vi "Autonomous Independent.vi"   [LabVIEW 2013]
doc: "This VI is called when autonomous begins, and will automatically be terminated when autonomous ends. You can carry out timed or sensor driven robot movement independently without needing to return to the caller."
uses:
  Robot Global Data.vi
  <vilib>/Rock Robotics/WPI/Joystick/WPI_JoystickGetSetRefNum.vi
types:
  T1 = typedef "WPI_DigitalInputDevRef.ctl" = cluster{"DevStatus":errorcluster, "DIO Channel":T2, "Digital Module":T3}
  T2 = typedef "FPGA_DIOChannel.ctl" = enum8{"DIO 1", "DIO 2", "DIO 3", "DIO 4", "DIO 5", "DIO 6", "DIO 7", "DIO 8", "DIO 9", "DIO 10", "DIO 11", "DIO 12", "DIO 13", "DIO 14", "Invalid"}
  T3 = typedef "FPGA_TypedefDigitalModule.ctl" = enum16{"Digital Module 1", "Digital Module 2"}
  T4 = typedef "WPI_MotorControlDeviceRef.ctl" = cluster{"DeviceStatus":errorcluster, "Type":enum16{"PWM", "CAN"}, "PWM":cluster{"Digital Module":T3, "PWM Channel":T5, "DeadBand":T6}, "CAN":cluster{"Device Number":u8, "Control Mode":T7, "Semaphore":T8, "Max Vout":dbl}, "Invert":bool, "TransformRef":T9, "InvTransformRef":T9}
  T5 = typedef "FPGA_DIOPWMChannel.ctl" = enum8{"PWM 1", "PWM 2", "PWM 3", "PWM 4", "PWM 5", "PWM 6", "PWM 7", "PWM 8", "PWM 9", "PWM 10", "Invalid"}
  T6 = typedef "WPI_PWMDeadband.ctl" = cluster{"Name":string, "maxPositivePwm":i32, "minPositivePwm":i32, "centerPwm":i32, "maxNegativePwm":i32, "minNegativePwm":i32, "angularRange":u16}
  T7 = typedef "WPI_CANJaguar_ControlMode.ctl" = enum8{"Percent VBus", "Current", "Speed", "Position", "Voltage"}
  T8 = typedef "Semaphore RefNum" = refnum<k1>
  T9 = typedef "WPI_PWMTransform_ConPane.ctl" = refnum<vi>
  T10 = typedef "WPI_JoystickDevRef.ctl" = cluster{"Device":T11}
  T11 = typedef "WPI_JoystickDeviceEnum.ctl" = enum16{"USB 1", "USB 2", "USB 3", "USB 4", "Kinect 1", "Kinect 2"}
  T12 = cluster{"axis 1 (x)":dbl, "axis 2 (y)":dbl, "axis 3 (throttle)":dbl, "axis 4":dbl, "axis 5":dbl, "axis 6":dbl}
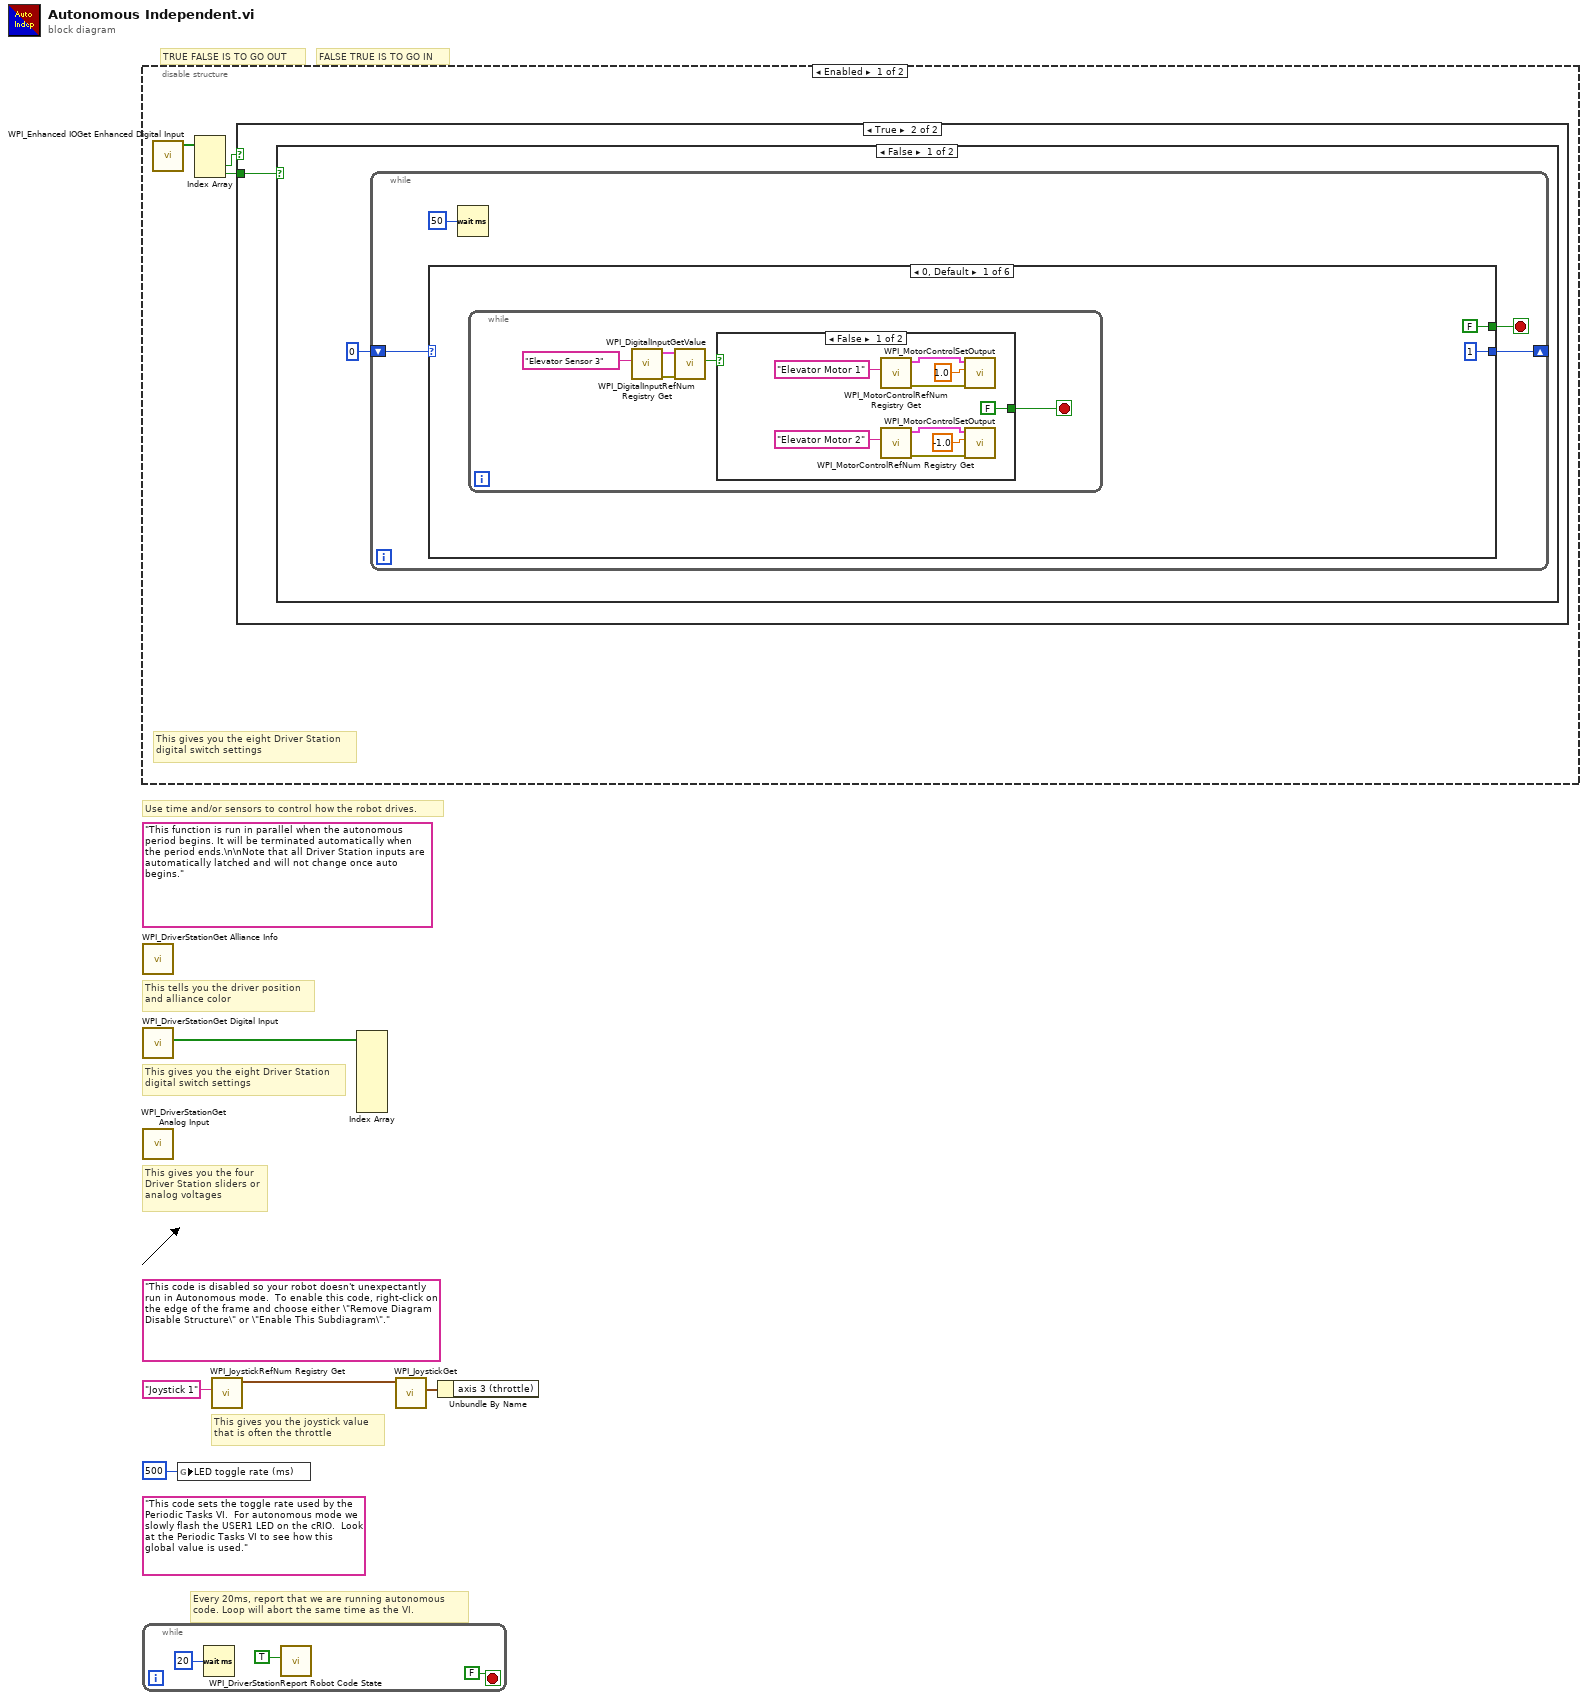
[diagram p0: block diagram]
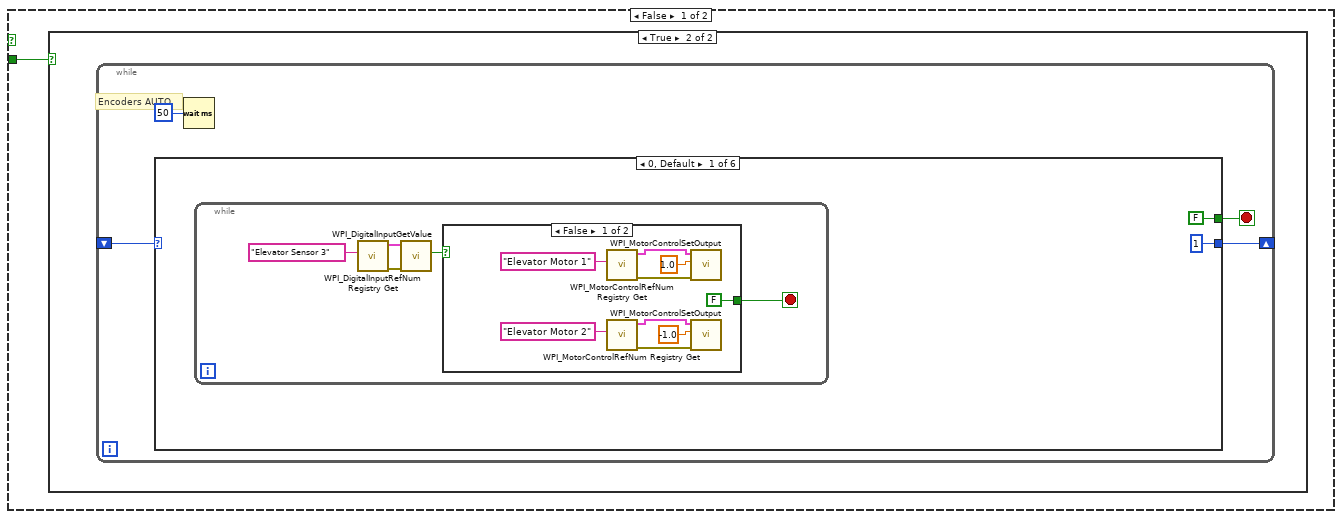
[diagram p2: hidden frame]
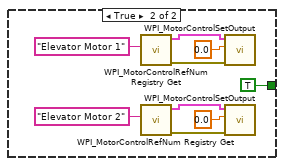
[diagram p4: hidden frame]
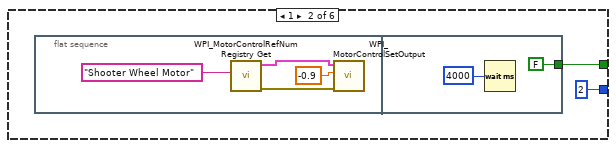
[diagram p5: hidden frame]
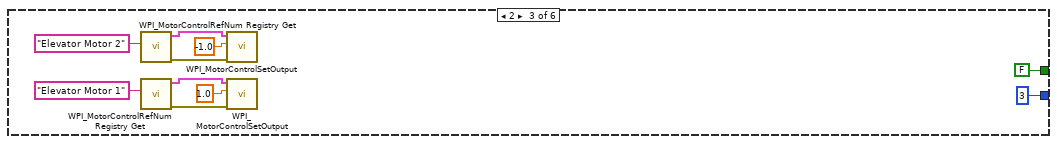
[diagram p6: hidden frame]
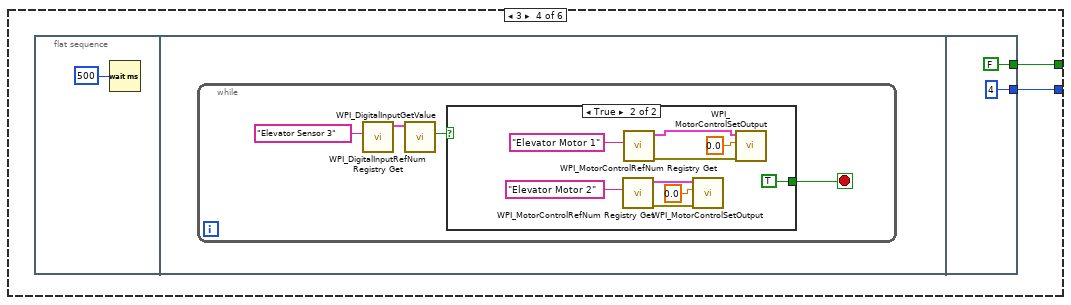
[diagram p7: hidden frame]
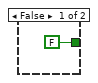
[diagram p8: hidden frame]
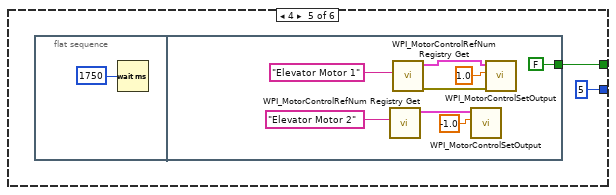
[diagram p9: hidden frame]
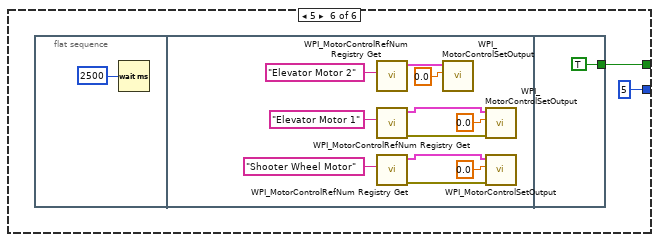
[diagram p10: hidden frame]
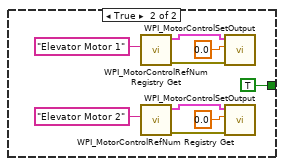
[diagram p11: hidden frame]
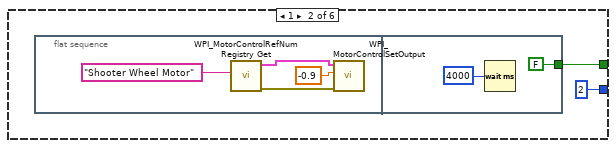
[diagram p12: hidden frame]
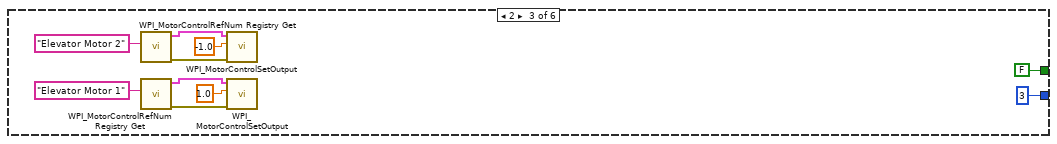
[diagram p13: hidden frame]
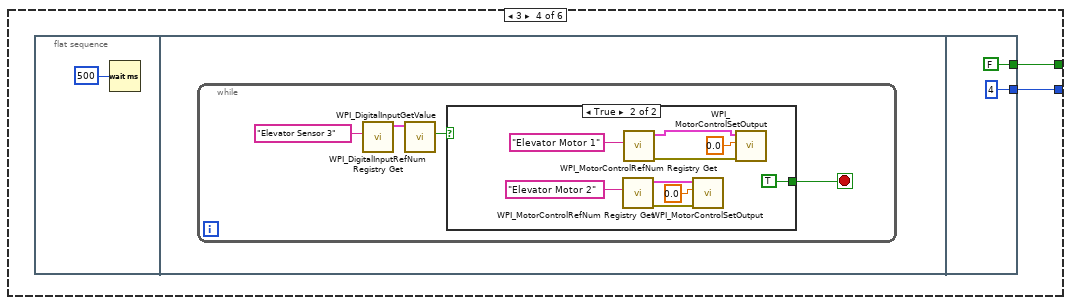
[diagram p14: hidden frame]
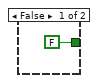
[diagram p15: hidden frame]
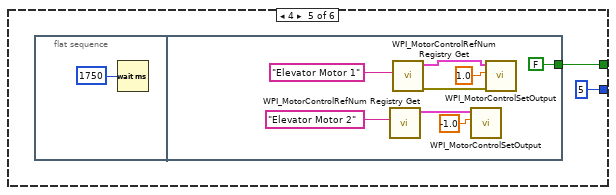
[diagram p16: hidden frame]
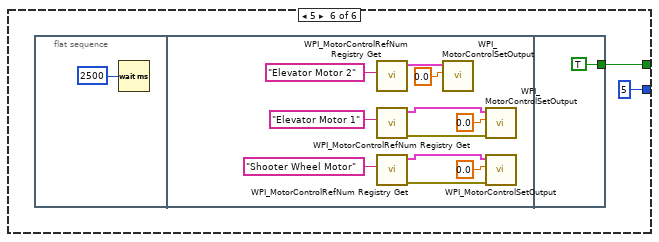
[diagram p17: hidden frame]
diagram:
  (unwired) "This code sets the toggle rate used by the Periodic Tasks VI.  For autonomous mode we slowly flash the USER1 LED on the cRIO.  Look at the Periodic Tasks VI to see how this global value is used."
  (unwired) "This code is disabled so your robot doesn't unexpectantly run in Autonomous mode.  To enable this code, right-click on the edge of the frame and choose either \"Remove Diagram Disable Structure\" or \"Enable This Subdiagram\"."
  (unwired) "This function is run in parallel when the autonomous period begins. It will be terminated automatically when the period ends.\n\nNote that all Driver Station inputs are automatically latched and will not change once auto begins."
  # "FALSE TRUE IS TO GO IN"
  # "TRUE FALSE IS TO GO OUT"
  # "Every 20ms, report that we are running autonomous\ncode. Loop will abort the same time as the VI."
  # "This gives you the joystick value\nthat is often the throttle"
  # "Use time and/or sensors to control how the robot drives."
  # "This tells you the driver position\nand alliance color"
  # "This gives you the eight Driver Station\ndigital switch settings"
  # "This gives you the four\nDriver Station sliders or\nanalog voltages"
  n1 = disable-structure shown="Enabled" {
    frame Enabled {
      # "This gives you the eight Driver Station\ndigital switch settings"
      n2 = call <vilib>:"WPI_Enhanced IOGet Enhanced Digital Input.vi"() -> ("Digital Input [1-16]"=w8:bool[])  [unwired: 10 in, 1 out]
      n3 = Index Array(array=w8) -> (element #2=w7:bool, element #3=w6:bool)  [unwired: 3 in, 1 out]
      n4 = case shown="True" w7 {
        tunnel: w6 -> [w9 w102]
        frame False {
          n5 = case shown="True" w9 {
            frame False {
            }
            frame True {
              # "Encoders AUTO"
              n6 = while {
                shift-right: [w11] -> _
                shift-left: _ -> [w10]
                stop <- w12 stop-if-true
                n7 = case shown="0, Default" w10 {
                  tunnel: [1 2 3 w57 5 5] -> w11
                  tunnel: [FALSE w39 FALSE w58 w76 w87] -> w12
                  frame 0, Default {
                    n8 = while {
                      stop <- w20 stop-if-true
                      n9 = call <vilib>:"WPI_DigitalInputRefNum Registry Get.vi"("refnum name"="Elevator Sensor 3") -> ("error out"=w19:errorcluster, "DigitalInputDevRef"=w18:T1)  [unwired: 9 in]
                      n10 = call <vilib>:"WPI_DigitalInputGetValue.vi"("error in (no error)"=w19, "DigitalInputDevRef"=w18) -> ("Value"=w16:bool)  [unwired: 7 in, 2 out]
                      n11 = case shown="False" w16 {
                        tunnel: [FALSE TRUE] -> w20
                        frame False {
                          n12 = call <vilib>:"WPI_MotorControlRefNum Registry Get.vi"("refnum name"="Elevator Motor 1") -> ("error out"=w26:errorcluster, "MotorControlDevRef"=w25:T4)  [unwired: 9 in]
                          n13 = call <vilib>:"WPI_MotorControlRefNum Registry Get.vi"("refnum name"="Elevator Motor 2") -> ("error out"=w29:errorcluster, "MotorControlDevRef"=w22:T4)  [unwired: 9 in]
                          n14 = call <vilib>:"WPI_MotorControlSetOutput.vi"("error in (no error)"=w26, "Output"=1.0, "MotorControlDevRef"=w25) -> ()  [unwired: 6 in, 3 out]
                          n15 = call <vilib>:"WPI_MotorControlSetOutput.vi"("error in (no error)"=w29, "Output"=-1.0, "MotorControlDevRef"=w22) -> ()  [unwired: 6 in, 3 out]
                        }
                        frame True {
                          n16 = call <vilib>:"WPI_MotorControlRefNum Registry Get.vi"("refnum name"="Elevator Motor 1") -> ("error out"=w35:errorcluster, "MotorControlDevRef"=w34:T4)  [unwired: 9 in]
                          n17 = call <vilib>:"WPI_MotorControlRefNum Registry Get.vi"("refnum name"="Elevator Motor 2") -> ("error out"=w38:errorcluster, "MotorControlDevRef"=w31:T4)  [unwired: 9 in]
                          n18 = call <vilib>:"WPI_MotorControlSetOutput.vi"("error in (no error)"=w35, "Output"=0.0, "MotorControlDevRef"=w34) -> ()  [unwired: 6 in, 3 out]
                          n19 = call <vilib>:"WPI_MotorControlSetOutput.vi"("error in (no error)"=w38, "Output"=0.0, "MotorControlDevRef"=w31) -> ()  [unwired: 6 in, 3 out]
                        }
                      }
                    }
                  }
                  frame 1 {
                    n20 = flat-sequence {
                      tunnel: [FALSE] -> w39
                      frame #0 {
                        n21 = call <vilib>:"WPI_MotorControlRefNum Registry Get.vi"("refnum name"="Shooter Wheel Motor") -> ("error out"=w44:errorcluster, "MotorControlDevRef"=w41:T4)  [unwired: 9 in]
                        n22 = call <vilib>:"WPI_MotorControlSetOutput.vi"("error in (no error)"=w44, "Output"=-0.9, "MotorControlDevRef"=w41) -> ()  [unwired: 6 in, 3 out]
                      }
                      frame #1 {
                        n23 = Wait (ms)(milliseconds to wait=u32 4000) -> ()  [unwired: 1 out]
                      }
                    }
                  }
                  frame 2 {
                    n24 = call <vilib>:"WPI_MotorControlRefNum Registry Get.vi"("refnum name"="Elevator Motor 2") -> ("error out"=w47:errorcluster, "MotorControlDevRef"=w48:T4)  [unwired: 9 in]
                    n25 = call <vilib>:"WPI_MotorControlRefNum Registry Get.vi"("refnum name"="Elevator Motor 1") -> ("error out"=w51:errorcluster, "MotorControlDevRef"=w52:T4)  [unwired: 9 in]
                    n26 = call <vilib>:"WPI_MotorControlSetOutput.vi"("error in (no error)"=w47, "Output"=-1.0, "MotorControlDevRef"=w48) -> ()  [unwired: 6 in, 3 out]
                    n27 = call <vilib>:"WPI_MotorControlSetOutput.vi"("error in (no error)"=w51, "Output"=1.0, "MotorControlDevRef"=w52) -> ()  [unwired: 6 in, 3 out]
                  }
                  frame 3 {
                    n28 = flat-sequence {
                      tunnel: [FALSE] -> w58
                      tunnel: [4] -> w57
                      frame #0 {
                        n29 = Wait (ms)(milliseconds to wait=u32 500) -> ()  [unwired: 1 out]
                      }
                      frame #1 {
                        n30 = while {
                          stop <- w60 stop-if-true
                          n31 = call <vilib>:"WPI_DigitalInputRefNum Registry Get.vi"("refnum name"="Elevator Sensor 3") -> ("DigitalInputDevRef"=w62:T1)  [unwired: 9 in, 1 out]
                          n32 = call <vilib>:"WPI_DigitalInputGetValue.vi"("DigitalInputDevRef"=w62) -> ("Value"=w61:bool)  [unwired: 8 in, 2 out]
                          n33 = case shown="True" w61 {
                            tunnel: [FALSE TRUE] -> w60
                            frame False {
                            }
                            frame True {
                              n34 = call <vilib>:"WPI_MotorControlRefNum Registry Get.vi"("refnum name"="Elevator Motor 2") -> ("error out"=w65:errorcluster, "MotorControlDevRef"=w67:T4)  [unwired: 9 in]
                              n35 = call <vilib>:"WPI_MotorControlRefNum Registry Get.vi"("refnum name"="Elevator Motor 1") -> ("error out"=w68:errorcluster, "MotorControlDevRef"=w69:T4)  [unwired: 9 in]
                              n36 = call <vilib>:"WPI_MotorControlSetOutput.vi"("error in (no error)"=w65, "Output"=0.0, "MotorControlDevRef"=w67) -> ()  [unwired: 6 in, 3 out]
                              n37 = call <vilib>:"WPI_MotorControlSetOutput.vi"("error in (no error)"=w68, "Output"=0.0, "MotorControlDevRef"=w69) -> ()  [unwired: 6 in, 3 out]
                            }
                          }
                        }
                      }
                      frame #2 {
                      }
                    }
                  }
                  frame 4 {
                    n38 = flat-sequence {
                      tunnel: [FALSE] -> w76
                      frame #0 {
                        n39 = Wait (ms)(milliseconds to wait=u32 1750) -> ()  [unwired: 1 out]
                      }
                      frame #1 {
                        n40 = call <vilib>:"WPI_MotorControlRefNum Registry Get.vi"("refnum name"="Elevator Motor 2") -> ("MotorControlDevRef"=w86:T4)  [unwired: 9 in, 1 out]
                        n41 = call <vilib>:"WPI_MotorControlRefNum Registry Get.vi"("refnum name"="Elevator Motor 1") -> ("error out"=w85:errorcluster, "MotorControlDevRef"=w79:T4)  [unwired: 9 in]
                        n42 = call <vilib>:"WPI_MotorControlSetOutput.vi"("Output"=-1.0, "MotorControlDevRef"=w86) -> ()  [unwired: 7 in, 3 out]
                        n43 = call <vilib>:"WPI_MotorControlSetOutput.vi"("error in (no error)"=w85, "Output"=1.0, "MotorControlDevRef"=w79) -> ()  [unwired: 6 in, 3 out]
                      }
                    }
                  }
                  frame 5 {
                    n44 = flat-sequence {
                      tunnel: [TRUE] -> w87
                      frame #0 {
                        n45 = Wait (ms)(milliseconds to wait=u32 2500) -> ()  [unwired: 1 out]
                      }
                      frame #1 {
                        n46 = call <vilib>:"WPI_MotorControlRefNum Registry Get.vi"("refnum name"="Elevator Motor 2") -> ("MotorControlDevRef"=w96:T4)  [unwired: 9 in, 1 out]
                        n47 = call <vilib>:"WPI_MotorControlRefNum Registry Get.vi"("refnum name"="Elevator Motor 1") -> ("error out"=w95:errorcluster, "MotorControlDevRef"=w90:T4)  [unwired: 9 in]
                        n48 = call <vilib>:"WPI_MotorControlRefNum Registry Get.vi"("refnum name"="Shooter Wheel Motor") -> ("error out"=w100:errorcluster, "MotorControlDevRef"=w97:T4)  [unwired: 9 in]
                        n49 = call <vilib>:"WPI_MotorControlSetOutput.vi"("Output"=0.0, "MotorControlDevRef"=w96) -> ()  [unwired: 7 in, 3 out]
                        n50 = call <vilib>:"WPI_MotorControlSetOutput.vi"("error in (no error)"=w95, "Output"=0.0, "MotorControlDevRef"=w90) -> ()  [unwired: 6 in, 3 out]
                        n51 = call <vilib>:"WPI_MotorControlSetOutput.vi"("error in (no error)"=w100, "Output"=0.0, "MotorControlDevRef"=w97) -> ()  [unwired: 6 in, 3 out]
                      }
                      frame #2 {
                      }
                    }
                  }
                }
                n52 = Wait (ms)(milliseconds to wait=u32 50) -> ()  [unwired: 1 out]
              }
            }
          }
        }
        frame True {
          n53 = case shown="False" w102 {
            frame False {
              n54 = while {
                shift-right: [w105] -> _
                shift-left: 0 -> [w104]
                stop <- w106 stop-if-true
                n55 = case shown="0, Default" w104 {
                  tunnel: [1 2 3 w151 5 5] -> w105
                  tunnel: [FALSE w133 FALSE w152 w170 w181] -> w106
                  frame 0, Default {
                    n56 = while {
                      stop <- w114 stop-if-true
                      n57 = call <vilib>:"WPI_DigitalInputRefNum Registry Get.vi"("refnum name"="Elevator Sensor 3") -> ("error out"=w113:errorcluster, "DigitalInputDevRef"=w112:T1)  [unwired: 9 in]
                      n58 = call <vilib>:"WPI_DigitalInputGetValue.vi"("error in (no error)"=w113, "DigitalInputDevRef"=w112) -> ("Value"=w110:bool)  [unwired: 7 in, 2 out]
                      n59 = case shown="False" w110 {
                        tunnel: [FALSE TRUE] -> w114
                        frame False {
                          n60 = call <vilib>:"WPI_MotorControlRefNum Registry Get.vi"("refnum name"="Elevator Motor 1") -> ("error out"=w120:errorcluster, "MotorControlDevRef"=w119:T4)  [unwired: 9 in]
                          n61 = call <vilib>:"WPI_MotorControlRefNum Registry Get.vi"("refnum name"="Elevator Motor 2") -> ("error out"=w123:errorcluster, "MotorControlDevRef"=w116:T4)  [unwired: 9 in]
                          n62 = call <vilib>:"WPI_MotorControlSetOutput.vi"("error in (no error)"=w120, "Output"=1.0, "MotorControlDevRef"=w119) -> ()  [unwired: 6 in, 3 out]
                          n63 = call <vilib>:"WPI_MotorControlSetOutput.vi"("error in (no error)"=w123, "Output"=-1.0, "MotorControlDevRef"=w116) -> ()  [unwired: 6 in, 3 out]
                        }
                        frame True {
                          n64 = call <vilib>:"WPI_MotorControlRefNum Registry Get.vi"("refnum name"="Elevator Motor 1") -> ("error out"=w129:errorcluster, "MotorControlDevRef"=w128:T4)  [unwired: 9 in]
                          n65 = call <vilib>:"WPI_MotorControlRefNum Registry Get.vi"("refnum name"="Elevator Motor 2") -> ("error out"=w132:errorcluster, "MotorControlDevRef"=w125:T4)  [unwired: 9 in]
                          n66 = call <vilib>:"WPI_MotorControlSetOutput.vi"("error in (no error)"=w129, "Output"=0.0, "MotorControlDevRef"=w128) -> ()  [unwired: 6 in, 3 out]
                          n67 = call <vilib>:"WPI_MotorControlSetOutput.vi"("error in (no error)"=w132, "Output"=0.0, "MotorControlDevRef"=w125) -> ()  [unwired: 6 in, 3 out]
                        }
                      }
                    }
                  }
                  frame 1 {
                    n68 = flat-sequence {
                      tunnel: [FALSE] -> w133
                      frame #0 {
                        n69 = call <vilib>:"WPI_MotorControlRefNum Registry Get.vi"("refnum name"="Shooter Wheel Motor") -> ("error out"=w138:errorcluster, "MotorControlDevRef"=w135:T4)  [unwired: 9 in]
                        n70 = call <vilib>:"WPI_MotorControlSetOutput.vi"("error in (no error)"=w138, "Output"=-0.9, "MotorControlDevRef"=w135) -> ()  [unwired: 6 in, 3 out]
                      }
                      frame #1 {
                        n71 = Wait (ms)(milliseconds to wait=u32 4000) -> ()  [unwired: 1 out]
                      }
                    }
                  }
                  frame 2 {
                    n72 = call <vilib>:"WPI_MotorControlRefNum Registry Get.vi"("refnum name"="Elevator Motor 2") -> ("error out"=w141:errorcluster, "MotorControlDevRef"=w142:T4)  [unwired: 9 in]
                    n73 = call <vilib>:"WPI_MotorControlRefNum Registry Get.vi"("refnum name"="Elevator Motor 1") -> ("error out"=w145:errorcluster, "MotorControlDevRef"=w146:T4)  [unwired: 9 in]
                    n74 = call <vilib>:"WPI_MotorControlSetOutput.vi"("error in (no error)"=w141, "Output"=-1.0, "MotorControlDevRef"=w142) -> ()  [unwired: 6 in, 3 out]
                    n75 = call <vilib>:"WPI_MotorControlSetOutput.vi"("error in (no error)"=w145, "Output"=1.0, "MotorControlDevRef"=w146) -> ()  [unwired: 6 in, 3 out]
                  }
                  frame 3 {
                    n76 = flat-sequence {
                      tunnel: [FALSE] -> w152
                      tunnel: [4] -> w151
                      frame #0 {
                        n77 = Wait (ms)(milliseconds to wait=u32 500) -> ()  [unwired: 1 out]
                      }
                      frame #1 {
                        n78 = while {
                          stop <- w154 stop-if-true
                          n79 = call <vilib>:"WPI_DigitalInputRefNum Registry Get.vi"("refnum name"="Elevator Sensor 3") -> ("DigitalInputDevRef"=w156:T1)  [unwired: 9 in, 1 out]
                          n80 = call <vilib>:"WPI_DigitalInputGetValue.vi"("DigitalInputDevRef"=w156) -> ("Value"=w155:bool)  [unwired: 8 in, 2 out]
                          n81 = case shown="True" w155 {
                            tunnel: [FALSE TRUE] -> w154
                            frame False {
                            }
                            frame True {
                              n82 = call <vilib>:"WPI_MotorControlRefNum Registry Get.vi"("refnum name"="Elevator Motor 2") -> ("error out"=w159:errorcluster, "MotorControlDevRef"=w161:T4)  [unwired: 9 in]
                              n83 = call <vilib>:"WPI_MotorControlRefNum Registry Get.vi"("refnum name"="Elevator Motor 1") -> ("error out"=w162:errorcluster, "MotorControlDevRef"=w163:T4)  [unwired: 9 in]
                              n84 = call <vilib>:"WPI_MotorControlSetOutput.vi"("error in (no error)"=w159, "Output"=0.0, "MotorControlDevRef"=w161) -> ()  [unwired: 6 in, 3 out]
                              n85 = call <vilib>:"WPI_MotorControlSetOutput.vi"("error in (no error)"=w162, "Output"=0.0, "MotorControlDevRef"=w163) -> ()  [unwired: 6 in, 3 out]
                            }
                          }
                        }
                      }
                      frame #2 {
                      }
                    }
                  }
                  frame 4 {
                    n86 = flat-sequence {
                      tunnel: [FALSE] -> w170
                      frame #0 {
                        n87 = Wait (ms)(milliseconds to wait=u32 1750) -> ()  [unwired: 1 out]
                      }
                      frame #1 {
                        n88 = call <vilib>:"WPI_MotorControlRefNum Registry Get.vi"("refnum name"="Elevator Motor 2") -> ("MotorControlDevRef"=w180:T4)  [unwired: 9 in, 1 out]
                        n89 = call <vilib>:"WPI_MotorControlRefNum Registry Get.vi"("refnum name"="Elevator Motor 1") -> ("error out"=w179:errorcluster, "MotorControlDevRef"=w173:T4)  [unwired: 9 in]
                        n90 = call <vilib>:"WPI_MotorControlSetOutput.vi"("Output"=-1.0, "MotorControlDevRef"=w180) -> ()  [unwired: 7 in, 3 out]
                        n91 = call <vilib>:"WPI_MotorControlSetOutput.vi"("error in (no error)"=w179, "Output"=1.0, "MotorControlDevRef"=w173) -> ()  [unwired: 6 in, 3 out]
                      }
                    }
                  }
                  frame 5 {
                    n92 = flat-sequence {
                      tunnel: [TRUE] -> w181
                      frame #0 {
                        n93 = Wait (ms)(milliseconds to wait=u32 2500) -> ()  [unwired: 1 out]
                      }
                      frame #1 {
                        n94 = call <vilib>:"WPI_MotorControlRefNum Registry Get.vi"("refnum name"="Elevator Motor 2") -> ("MotorControlDevRef"=w190:T4)  [unwired: 9 in, 1 out]
                        n95 = call <vilib>:"WPI_MotorControlRefNum Registry Get.vi"("refnum name"="Elevator Motor 1") -> ("error out"=w189:errorcluster, "MotorControlDevRef"=w184:T4)  [unwired: 9 in]
                        n96 = call <vilib>:"WPI_MotorControlRefNum Registry Get.vi"("refnum name"="Shooter Wheel Motor") -> ("error out"=w194:errorcluster, "MotorControlDevRef"=w191:T4)  [unwired: 9 in]
                        n97 = call <vilib>:"WPI_MotorControlSetOutput.vi"("Output"=0.0, "MotorControlDevRef"=w190) -> ()  [unwired: 7 in, 3 out]
                        n98 = call <vilib>:"WPI_MotorControlSetOutput.vi"("error in (no error)"=w189, "Output"=0.0, "MotorControlDevRef"=w184) -> ()  [unwired: 6 in, 3 out]
                        n99 = call <vilib>:"WPI_MotorControlSetOutput.vi"("error in (no error)"=w194, "Output"=0.0, "MotorControlDevRef"=w191) -> ()  [unwired: 6 in, 3 out]
                      }
                      frame #2 {
                      }
                    }
                  }
                }
                n100 = Wait (ms)(milliseconds to wait=u32 50) -> ()  [unwired: 1 out]
              }
            }
            frame True {
            }
          }
        }
      }
    }
    frame Disabled {
    }
  }
  n101 = call <vilib>:"WPI_DriverStationGet Alliance Info.vi"() -> ()  [unwired: 12 out]
  n102 = call <vilib>:"WPI_DriverStationGet Digital Input.vi"() -> ("Driver Station Digital Input (1-8)"=w5:bool[])  [unwired: 11 out]
  n103 = call <vilib>:"WPI_DriverStationGet Analog Input.vi"() -> ()  [unwired: 12 out]
  n104 = while {
    stop <- FALSE stop-if-true
    n105 = Wait (ms)(milliseconds to wait=u32 20) -> ()  [unwired: 1 out]
    n106 = call <vilib>:"WPI_DriverStationReport Robot Code State.vi"("Autonomous"=TRUE) -> ()  [unwired: 10 in, 1 out]
  }
  n107 = global write "Robot Global Data.vi" "LED toggle rate (ms)"(u32 500 ("LED ms toggle rate")) -> ()
  n108 = call <vilib>:"WPI_JoystickRefNum Registry Get.vi"("refnum name"="Joystick 1") -> ("JoystickDevRef"=w2:T10)  [unwired: 1 in, 9 out]
  n109 = Index Array(array=w5) -> ()  [unwired: 8 in, 8 out]
  n110 = call <vilib>:"WPI_JoystickGet.vi"("JoystickDevRef"=w2) -> ("Axes"=w3:T12)  [unwired: 1 in, 5 out]
  n111 = Unbundle By Name(w3) -> ()  [unwired: 1 out]
